vi "Send message to Message Panel (and wait for response).vi"(0 "Prompt":string, 1 "Wait for response?":bool, 2 "Yes text":string, 3 "No text":string, 4 "Timeout?":bool) -> (5 "Response":bool)   [LabVIEW 2011]
panel:
  out "call chain":string[](array[string])
  in  "stop":bool
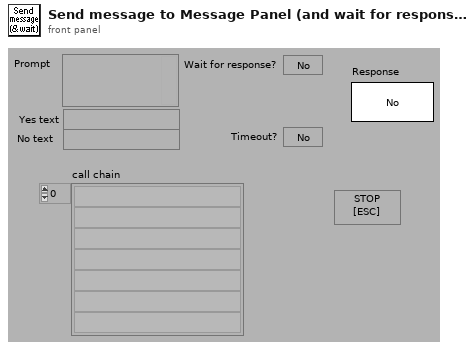
[diagram p1: front panel]
types:
  T1 = enum32{"Bad", "Idle", "Run top level", "Running"}
  T2 = enum16{"Initialise", "Add", "Check for response & remove"}
  T3 = cluster{"result string":string, "Yes text":string, "No text":string, "Timeout?":bool, bool, string, bool, bool, dbl}
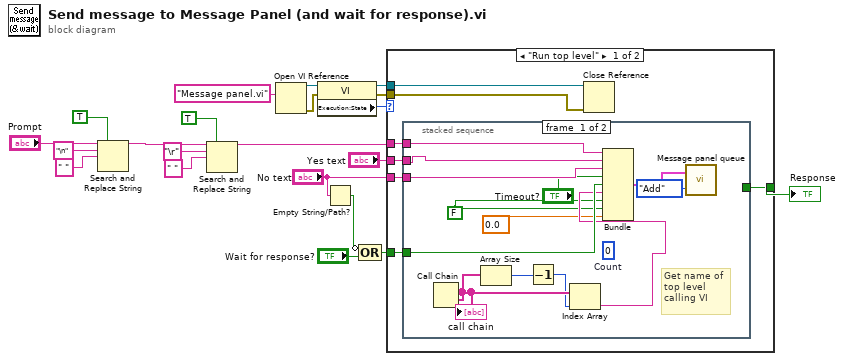
[diagram p0: block diagram]
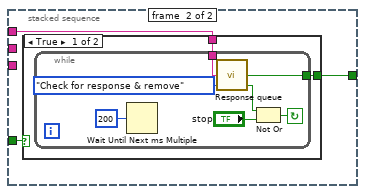
[diagram p2: hidden frame]
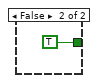
[diagram p3: hidden frame]
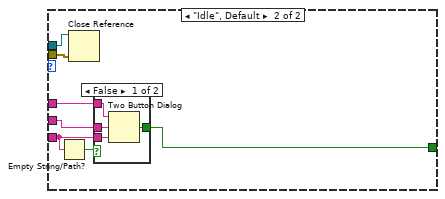
[diagram p4: hidden frame]
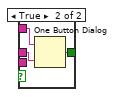
[diagram p5: hidden frame]
diagram:
  n1 = Search and Replace String(replace all?=TRUE ("replace all? (F)"), input string="Prompt", search string="\n", replace string=" " ("replace string (\"\")")) -> (result string=w2:string)  [unwired: 4 in, 3 out]
  n2 = Search and Replace String(replace all?=TRUE ("replace all? (F)"), input string=w2, search string="\r", replace string=" " ("replace string (\"\")")) -> (result string=w1:string)  [unwired: 4 in, 3 out]
  n3 = Open VI Reference(vi path="Message panel.vi") -> (vi reference=w21:refnum<vi>, error out=w19:errorcluster)  [unwired: 5 in]
  n4 = property class="VI"(reference=w21, error in=w19) -> (reference out=w16:refnum<vi>, error out=w15:errorcluster, "Execution:State"=w17:T1)
  n5 = Empty String/Path?(string/path="No text") -> (empty?=w11:bool)
  n6 = Compound Arithmetic op=OR(invert w11, "Wait for response?") -> (w12:bool)
  n7 = case shown="\"Run top level\"" w17 {
    tunnel: [w28 w55] -> w18
    tunnel: w16 -> [w23 w61]
    tunnel: w15 -> [w22 w60]
    tunnel: w1 -> [w27 w57]
    tunnel: "Yes text" -> [w26 w58]
    tunnel: "No text" -> [w25 w59]
    tunnel: w12 -> [w24 _]
    frame "Run top level" {
      n8 = stacked-sequence {
        tunnel: [_ w44] -> w28
        tunnel: w27 -> [w31 w43]
        tunnel: w26 -> [w39 _]
        tunnel: w25 -> [w38 _]
        tunnel: w24 -> [w36 w42]
        frame #0 {
          w29 = FALSE
          (unwired) 0  # Count
          # "Get name of\ntop level\ncalling VI"
          n9 = Call Chain() -> (call chain=w35:string[])
          "call chain" <- w35
          n10 = Array Size(array=w35) -> (size(s)=w34:i32)
          n11 = Decrement(x=w34) -> (x-1=w33:i32)
          n12 = Index Array(array=w35, index=w33) -> (element=w32:string)
          n13 = Bundle("result string"=w31, "Yes text"=w39, "No text"=w38, "Timeout?"="Timeout?", w36, w32, w29, w29, 0.0) -> (w40:T3)  [unwired: 1 in]
          n14 = call "Message panel queue.vi"("Action"=enum16{"Initialise", "Add", "Read (& remove)"}."Add", "New item"=w40) -> ()  [unwired: 1 in, 1 out]
        }
        frame #1 {
          n15 = case shown="True" w42 {
            tunnel: [w46 TRUE ("Response")] -> w44
            tunnel: w43 -> [w45 _]
            frame True {
              n16 = while {
                tunnel: w45 -> [w47]
                tunnel: [w49] -> w46
                stop <- w50 continue-if-true
                n17 = Wait Until Next ms Multiple(millisecond multiple=u32 200) -> ()  [unwired: 1 out]
                n18 = call "Response queue.vi"("Action"=T2."Check for response & remove", "Prompt of item possibly in queue"=w47) -> ("Item present (& removed)?"=w51:bool, "Response"=w49:bool)  [unwired: 2 in]
                n19 = Not Or(1:"stop", 2:w51) -> (0:w50:bool)
              }
            }
            frame False {
            }
          }
        }
      }
      n20 = Close Reference(reference=w23, error in (no error)=w22) -> ()  [unwired: 1 out]
    }
    frame "Idle", Default {
      n21 = Empty String/Path?(string/path=w59) -> (empty?=w56:bool)
      n22 = Close Reference(reference=w61, error in (no error)=w60) -> ()  [unwired: 1 out]
      n23 = case shown="False" w56 {
        tunnel: [w65 w67] -> w55
        tunnel: w58 -> [w64 w66]
        tunnel: w59 -> [w63 _]
        tunnel: w57 -> [w62 w68]
        frame False {
          n24 = Two Button Dialog(message=w62, 1:w63, 2:w64) -> (T button?=w65:bool)
        }
        frame True {
          n25 = One Button Dialog(message=w68, button name ("OK")=w66) -> (true=w67:bool)
        }
      }
    }
  }
  "Response" <- w18
